vi "FTW-Logger-Construct.vi"(0 "Initialization Sequence":string, 5 "Logger Configuration":T1, 11 "error in":errorcluster) -> (4 "FTW Logger":refnum<class "FTW-Logger-Core.lvclass">, 6 "Incoming Requests":refnum<event-registration>, 15 "error out":errorcluster)   [LabVIEW 2012, in "FTW-Actor.lvlib" / "FTW-Logger-Core.lvclass"]
uses:
  FTW-Logger-Core.lvclass
  Utility/FTW-Actor-Configuration.ctl
  Message/Request/FTW-Message-IncomingRequest.lvclass
  FTW-Logger-Core.lvclass/FTW-Logger-Core.ctl
  Core/src/JSON/FTW-JSON-RegexParse.vi
  Core/src/Regex/FTW-Regex.vi
  Core/src/JSON/FTW-JSON-RegexHeader.vi
  Core/src/Error/FTW-ERR-ThrowError.vi
  Core/src/Error/FTW-ERR-ThrowGenericError.vi
  Core/src/Container/FTW-Container-Construct.vi
  Core/src/Container/FTW-Container-Load-JSON.vi
  Core/src/Container/FTW-Container-Destroy.vi
  Core/utils/CodeGen/JSON Deserialize/FTW-JSON-Deserialize.xnode
  Core/src/Container/FTW-Container.lvclass
  FTW-Actor.lvlib
panel:
  # "Inputs"
  # "Outputs"
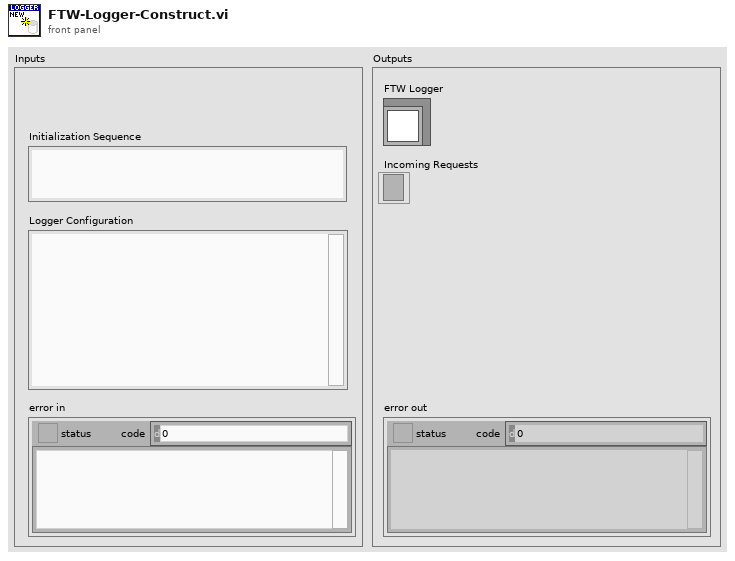
[diagram p1: front panel]
types:
  T1 = typedef "FTW-Actor.lvlib/FTW-Actor-Configuration.ctl" = string
  T2 = cluster{"LoggerDirectory":path, "LoggerDiskThrashDelay":u32, "LoggerID":string, "ApplicationName":string}
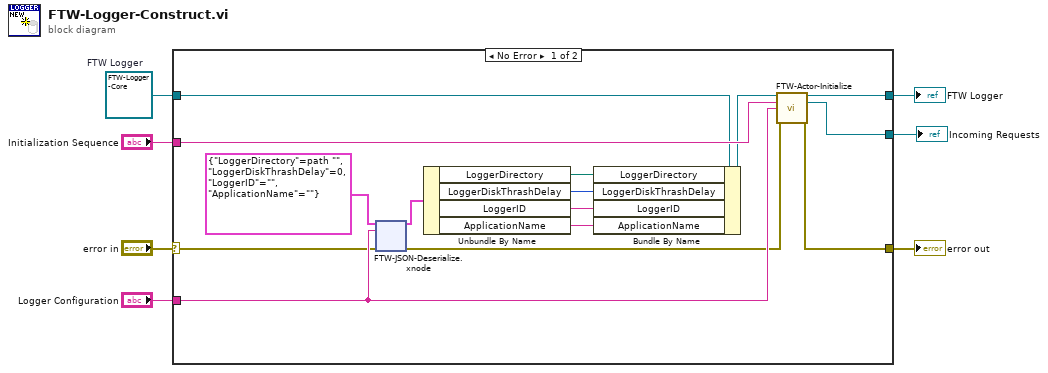
[diagram p0: block diagram]
diagram:
  w7 = refnum<class "FTW-Logger-Core.lvclass"> refnum  # FTW Logger
  n1 = case shown="No Error" "error in" {
    selector: "error in" -> [w9 w57]
    tunnel: [w20 w57] -> w5
    tunnel: [w22 w56] -> w1
    tunnel: w7 -> [w18 w56]
    tunnel: "Logger Configuration" -> [w10 _]
    tunnel: [w21 _] -> w3
    tunnel: "Initialization Sequence" -> [w19 _]
    frame No Error {
      n2 = xnode "FTW-JSON-Deserialize.xnode"("Data Type and Default Values"=T2 {"LoggerDirectory"=path "", "LoggerDiskThrashDelay"=0, "LoggerID"="", "ApplicationName"=""}, "JSON String"=w10, "error in"=w9) -> ("Populated Values"=w11:T2, "error out"=w8:errorcluster)
      n3 = Unbundle By Name(w11) -> ("LoggerDirectory"=w16:path, "LoggerDiskThrashDelay"=w15:u32, "LoggerID"=w14:string, "ApplicationName"=w13:string)
      n4 = Bundle By Name(cluster=w18, "LoggerDirectory"=w16, "LoggerDiskThrashDelay"=w15, "LoggerID"=w14, "ApplicationName"=w13) -> (w17:refnum<class "FTW-Logger-Core.lvclass">)
      n5 = call-dynamic "FTW-Actor-Initialize.vi"("FTW Actor Instance Type"=w17, "Initialization Job Sequence"=w19, "Actor Instance Configuration"=w10, "error in"=w8) -> ("FTW Actor Instance"=w22:refnum<class "FTW-Logger-Core.lvclass">, "Incoming Requests"=w21:refnum<event-registration>, "error out"=w20:errorcluster)  [unwired: 9 in]
    }
    frame Error {
    }
  }
  "error out" <- w5
  "FTW Logger" <- w1
  "Incoming Requests" <- w3
